vi "pruebaRapidaW&R.vi"() -> ()   [LabVIEW 2019]
uses:
  <vilib>/Instr/_visa.llb/VISA Configure Serial Port (Instr).vi
  <vilib>/Utility/error.llb/Error Cluster From Error Code.vi
  <vilib>/ErrorRing/Error Ring.xnode
panel:
  out "return count":u32
  out "read buffer":string
  out "x = y?":bool
  out "error out":errorcluster
  out "concatenated string":string
  out "PARAMETROS DE ENTRADA 2":T1={"Bandeja Origen"="BANDEJA OK", "Bandeja destino"="BANDEJA NOK", "NUMERO DE ASICS A MOVER"=0, " COORD.ORIGEN X"="00", "COORD.ORIGEN Y"="00", "COORD.DESTINO X"="00", "COORD. DESTINO Y"="00"}
  out "error IO":errorcluster
  in  "PARAMETROS DE ENTRADA":T1={"Bandeja Origen"="BANDEJA OK", "Bandeja destino"="BANDEJA NOK", "NUMERO DE ASICS A MOVER"=1, " COORD.ORIGEN X"="00", "COORD.ORIGEN Y"="00", "COORD.DESTINO X"="00", "COORD. DESTINO Y"="00"}
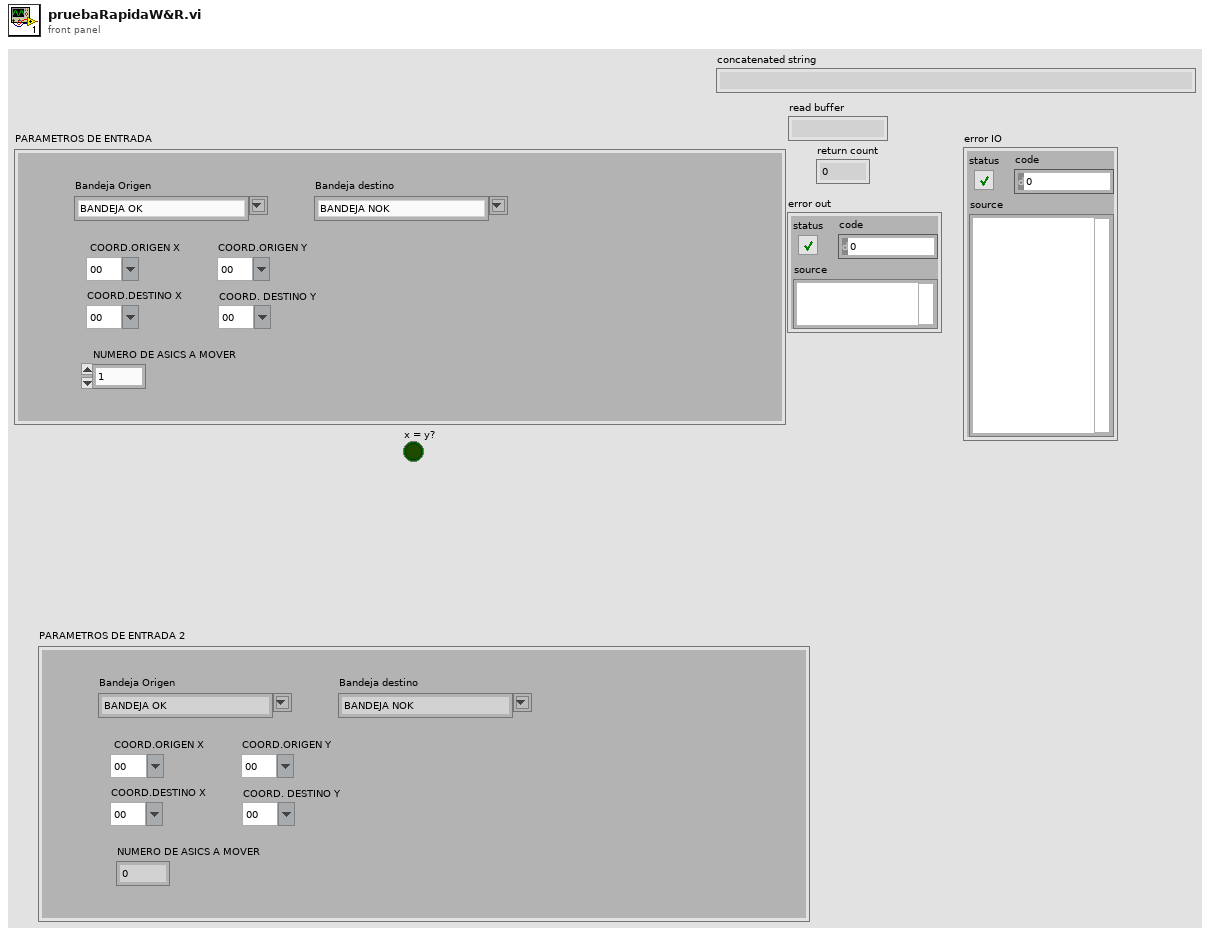
[diagram p1: front panel]
types:
  T1 = typedef "PARÁMETROS.ctl" = cluster{"Bandeja Origen":string, "Bandeja destino":string, "NUMERO DE ASICS A MOVER":i16, " COORD.ORIGEN X":string, "COORD.ORIGEN Y":string, "COORD.DESTINO X":string, "COORD. DESTINO Y":string}
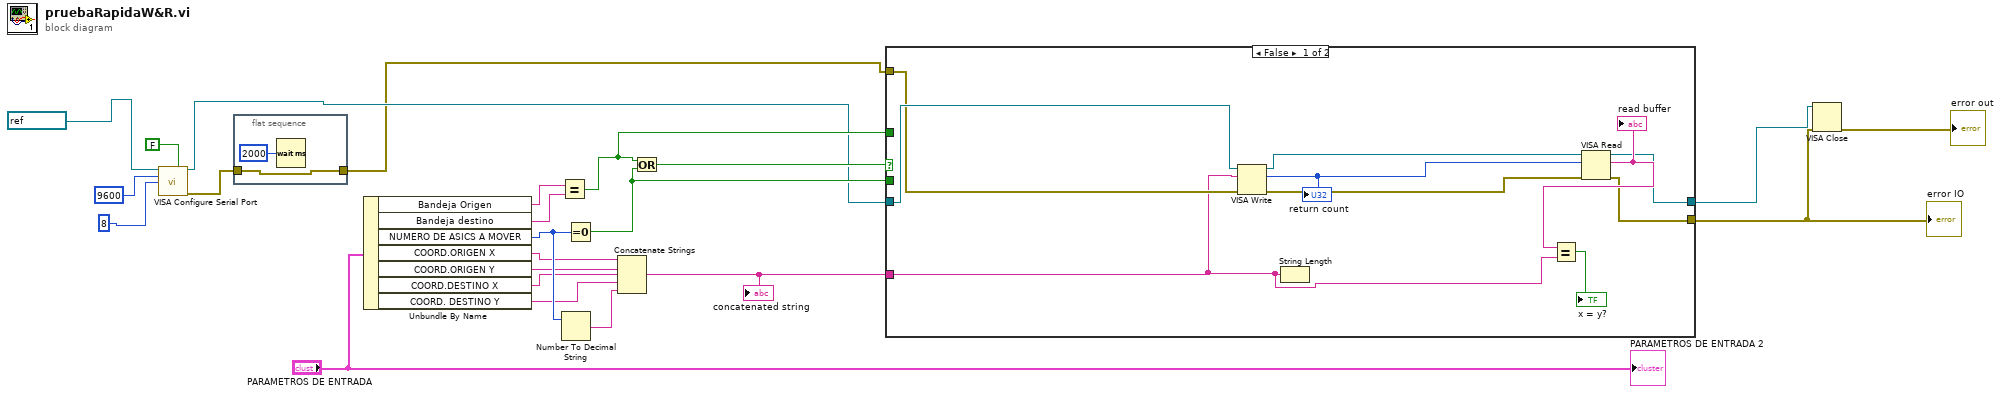
[diagram p0: block diagram]
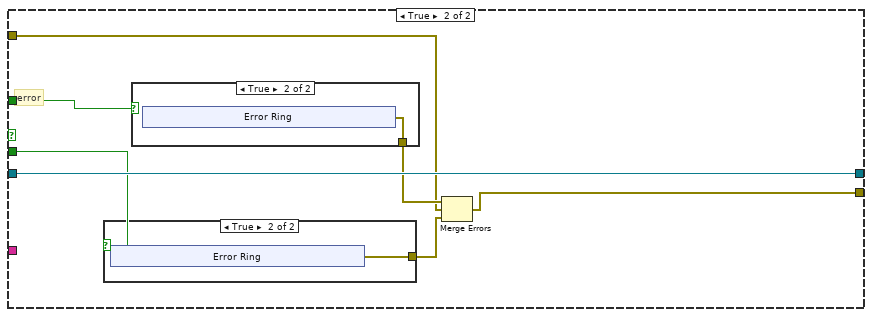
[diagram p2: hidden frame]
diagram:
  n1 = call-poly "VISA Configure Serial Port"("VISA resource name"=refnum<visa-resource-name> "COM5", "Enable Termination\nChar (T)"=FALSE ("Enable Termination\nChar (T)"), "baud rate (9600)"=u32 9600, "data bits (8)"=u16 8) -> ("VISA resource name out"=w14:refnum<visa-resource-name>, "error out"=w3:errorcluster)  [unwired: 10 in]
  n2 = flat-sequence {
    tunnel: w3 -> [w25]
    tunnel: [w25] -> w2
    frame #0 {
      n3 = Wait (ms)(milliseconds to wait=u32 2000) -> ()  [unwired: 1 out]
    }
  }
  n4 = Unbundle By Name("PARAMETROS DE ENTRADA") -> ("Bandeja Origen"=w19:string, "Bandeja destino"=w18:string, "NUMERO DE ASICS A MOVER"=w17:i16, "COORD.ORIGEN X"=w11:string, "COORD.ORIGEN Y"=w10:string, "COORD.DESTINO X"=w9:string, "COORD. DESTINO Y"=w1:string)
  n5 = Equal?(x=w19, y=w18) -> (x = y?=w21:bool)
  n6 = Number To Decimal String(number=w17) -> (decimal integer string=w8:string)  [unwired: 1 in]
  n7 = Equal To 0?(x=w17) -> (x = 0?=w20:bool)
  n8 = Concatenate Strings(w11, w10, w9, w1, w8) -> (w7:string)
  "concatenated string" <- w7
  n9 = Or(x=w21, y=w20) -> (x .or. y?=w22:bool)
  n10 = case shown="False" w22 {
    tunnel: [w33 w41] -> w5
    tunnel: w14 -> [w35 w42]
    tunnel: [w32 w42] -> w6
    tunnel: w21 -> [_ w40]
    tunnel: w20 -> [_ w39]
    tunnel: w7 -> [w29 _]
    tunnel: w2 -> [w30 w36]
    frame False {
      n11 = VISA Write(VISA resource name=w35, write buffer=w29, error in (no error)=w30) -> (VISA resource name out=w28:refnum<visa-resource-name>, return count=w27:u32, error out=w26:errorcluster)
      "return count" <- w27
      n12 = String Length(string=w29) -> ()  [unwired: 1 out]
      n13 = VISA Read(VISA resource name=w28, byte count=w27, error in (no error)=w26) -> (VISA resource name out=w32:refnum<visa-resource-name>, read buffer=w34:string, error out=w33:errorcluster)  [unwired: 1 out]
      "read buffer" <- w34
      n14 = Equal?(x=w34, y=w29) -> (x = y?=→"x = y?":bool)
    }
    frame True {
      # "error"
      n15 = case shown="True" w39 {
        tunnel: [_ w43] -> w37
        frame False {
        }
        frame True {
          n16 = xnode "Error Ring"() -> ("error out"=w43:errorcluster)
        }
      }
      n17 = case shown="True" w40 {
        tunnel: [_ w49] -> w38
        frame False {
        }
        frame True {
          n18 = xnode "Error Ring"() -> ("error out"=w49:errorcluster)
        }
      }
      n19 = Merge Errors(w38, w36, w37) -> (w41:errorcluster)
    }
  }
  "error IO" <- w5
  n20 = VISA Close(VISA resource name=w6, error in (no error)=w5) -> (error out=→"error out":errorcluster)
  "PARAMETROS DE ENTRADA 2" <- "PARAMETROS DE ENTRADA"
